vi "CAN Talon Position Control Pot.vi"() -> ()   [LabVIEW 2015]
uses:
  <vilib>/Rock Robotics/WPI/CAN/TalonSRX/WPI_CANTalonSRX_APIControlMode.ctl
  <vilib>/Rock Robotics/WPI/CAN/TalonSRX/WPI_CANTalonSRX_APIFeedbackSelect.ctl
  <vilib>/Rock Robotics/WPI/MotorControl/WPI_MotorControlOpenCANTalonSRX.vi
panel:
  in  "I":dbl
  in  "F":dbl=0.01
  in  "D":dbl
  in  "P":dbl=1.0
  in  "Master Device Number":u8
  in  "stop":bool
  out "Actual Pos":dbl
  out "Feedback Chart":cluster{dbl, dbl}(graph)
  in  "Target Pos":dbl
  out "Boolean":bool
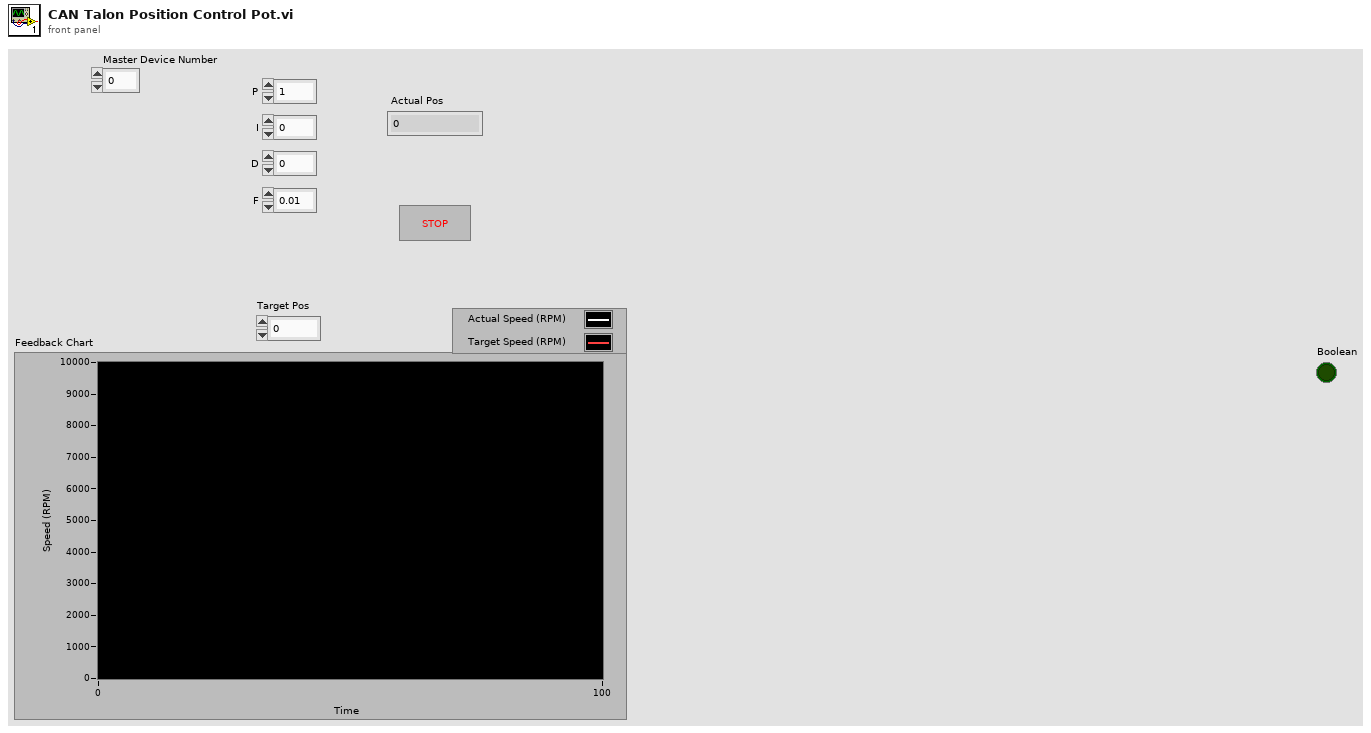
[diagram p1: front panel]
types:
  T1 = typedef "WPI_CANTalonSRX_APIFeedbackSelect.ctl" = enum16{"Digital Quadrature Encoder", "Analog Potentiometer", "Analog Encoder", "Count on Quad-A (Rising-Edge)", "Count on Quad-A (Falling-Edge)", "CTR Magnetic Enc (Absolute)", "CTR Magnetic Enc (Relative)", "Pulse Width"}
  T2 = typedef "WPI_CANTalonSRX_APIControlMode.ctl" = enum8{"Percent VBus", "Speed", "Position", "Slave", "Unchanged / Invalid", "Voltage Compensation", "Current", "Motion Profile"}
  T3 = typedef "WPI_MotorControlDeviceRef.ctl" = cluster{"DeviceStatus":errorcluster, "Type":T4, "PWM":cluster{"PWM Channel":T5, "DeadBand":T6}, "CAN":cluster{"Device Number":u8, "Control Mode":T7, "Semaphore":T8, "Max Vout":dbl, "TalonSRX Control Mode":T2}, "Invert":bool}
  T4 = typedef "WPI_MotorControlType.ctl" = enum16{"PWM", "CAN", "CANTalonSRX"}
  T5 = typedef "FPGA_DIOPWMChannel.ctl" = enum8{"PWM 0", "PWM 1", "PWM 2", "PWM 3", "PWM 4", "PWM 5", "PWM 6", "PWM 7", "PWM 8", "PWM 9", "PWM MXP 0", "PWM MXP 1", "PWM MXP 2", "PWM MXP 3", "PWM MXP 4", "PWM MXP 5", "PWM MXP 6", "PWM MXP 7", "PWM MXP 8", "PWM MXP 9", "Invalid"}
  T6 = typedef "WPI_PWMDeadband.ctl" = cluster{"Name":string, "maxPositivePwm":i32, "minPositivePwm":i32, "centerPwm":i32, "maxNegativePwm":i32, "minNegativePwm":i32, "angularRange":u16}
  T7 = typedef "WPI_CANJaguar_ControlMode.ctl" = enum8{"Percent VBus", "Current", "Speed", "Position", "Voltage"}
  T8 = typedef "Semaphore RefNum" = refnum<k1>
  T9 = typedef "WPI_CANTalonSRX_GlobalStatus.ctl" = cluster{"Applied Throttle":dbl, "Module Enabled":bool, "CAN Error":errorcluster, "Closed Loop Error":dbl, "Forward Limit Switch Closed":bool, "Reverse Limit Switch Closed":bool, "Sensor Position":dbl, "Sensor Velocity":dbl, "Current":dbl, "Sticky Fault - Over Temp":bool, "Sticky Fault - Under Voltage":bool, "Sticky Fault - Forward Limit":bool, "Sticky Fault - Reverse Limit":bool, "Sticky Fault - Forward Soft Limit":bool, "Sticky Fault - Reverse Soft Limit":bool, "Brake is Enabled":bool, "Encoder Position":dbl, "Encoder Velocity":dbl, "Encoder Index Count":dbl, "Encoder A Pin State":bool, "Encoder B Pin State":bool, "Encoder Index Pin State":bool, "Analog In":dbl, "Analog In Velocity":dbl, "Temperature (C)":dbl, "Battery Voltage":dbl, "Control 5 Is Supported":bool, "Current Profile Slot Select":dbl, "Pos Div 8":bool, "Vel Div 4":bool, "Pulse Width Position":i32, "Pulse Width Velocity":i32, "Pulse Width Rise To Rise (us)":i32, "Pulse Width Rise To Fall (us)":i32, "Mot Prof Active Is Under Run":bool, "Mot Prof Active Has Under Run":bool, "Mot Prof Active Is Last":bool, "Mot Prof Active Velocity Only":bool, "Mot Prof Active Is Valid":bool, "Mot Prof Buffer Is Full":bool, "Mot Prof Active Profile Slot Select":i32, "Mot Prof NextID":i32, "Mot Prof Count":i32, "Mot Prof Active Velocity":dbl, "Mot Prof Active Position":dbl, "Mot Prof Output Enable":i32}
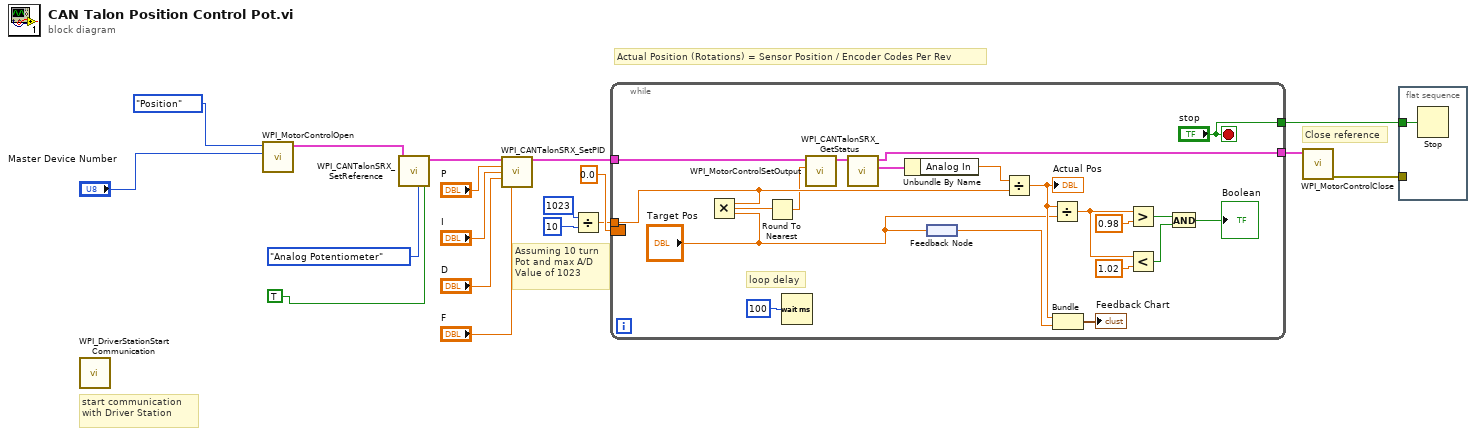
[diagram p0: block diagram]
diagram:
  # "Assuming 10 turn\nPot and max A/D\nValue of 1023"
  # "Actual Position (Rotations) = Sensor Position / Encoder Codes Per Rev"
  # "start communication with Driver Station"
  # "Close reference"
  n1 = call <vilib>:"WPI_DriverStationStart Communication.vi"() -> ()  [unwired: 2 in, 10 out]
  n2 = call-poly <vilib>:"WPI_MotorControlOpen.vi"("Device Number"="Master Device Number", "Control Mode"=WPI_CANTalonSRX_APIControlMode."Position") -> ("MotorControlDeviceRef"=w9:T3)  [unwired: 3 in, 6 out]
  n3 = call <vilib>:"WPI_CANTalonSRX_SetReference.vi"("Reverse Feedback Sensor"=TRUE, "Feedback Reference"=WPI_CANTalonSRX_APIFeedbackSelect."Analog Potentiometer", "CAN Talon SRX Ref"=w9) -> ("CAN Talon SRX Ref"=w8:T3)  [unwired: 7 in, 1 out]
  n4 = call <vilib>:"WPI_CANTalonSRX_SetPID.vi"("CAN Talon SRX Ref"=w8, "P"="P", "I"="I", "D"="D", "F"="F") -> ("CAN Talon SRX Ref"=w3:T3)  [unwired: 9 in, 1 out]
  n5 = Divide(x=1023, y=10) -> (x/y=w4:dbl)
  n6 = while {
    tunnel: ["stop"] -> w17
    tunnel: w3 -> [w30]
    tunnel: [w36] -> w18
    border: 0.0 -> [_]
    tunnel: w4 -> [w29]
    stop <- "stop" stop-if-true
    # "loop delay"
    n7 = Multiply(x=w29, y="Target Pos") -> (x*y=w20:dbl)
    n8 = Round To Nearest(number=w20) -> (nearest integer value=w19:dbl)
    n9 = Wait (ms)(milliseconds to wait=u32 100) -> ()  [unwired: 1 out]
    n10 = call <vilib>:"WPI_MotorControlSetOutput.vi"("Output"=w19, "MotorControlDevRef"=w30) -> ("MotorControlDevRef"=w35:T3)  [unwired: 7 in, 2 out]
    n11 = call <vilib>:"WPI_CANTalonSRX_GetStatus.vi"("CAN Talon SRX Ref"=w35) -> ("Talon SRX Status"=w34:T9, "CAN Talon SRX Ref"=w36:T3)  [unwired: 8 in, 1 out]
    n12 = Unbundle By Name(w34) -> ("Analog In"=w33:dbl)
    n13 = feedback #1() -> (w32:dbl)
    n14 = feedback-in #1("Target Pos") -> ()
    n15 = Divide(x=w33, y=w29) -> (x/y=w28:dbl)
    "Actual Pos" <- w28
    n16 = Divide(x=w28, y="Target Pos") -> (x/y=w26:dbl)
    n17 = Bundle(w28, w32) -> (→"Feedback Chart":cluster{dbl, dbl})  [unwired: 1 in]
    n18 = Greater?(x=w26, y=0.98) -> (0:w23:bool)
    n19 = Less?(x=w26, y=1.02) -> (x < y?=w22:bool)
    n20 = And(x=w23, y=w22) -> (x .and. y?=→"Boolean":bool)
  }
  n21 = call <vilib>:"WPI_MotorControlClose.vi"("MotorControlDevRef"=w18) -> ("error out"=w16:errorcluster)  [unwired: 10 in]
  n22 = flat-sequence {
    tunnel: w17 -> [w39]
    tunnel: w16 -> [_]
    frame #0 {
      n23 = Stop(stop? (T)=w39) -> ()
    }
  }
